vi "Create Queue.vi"(9 "Queue":refnum<class "Queue.lvclass">, 10 "Self Queue Alias":string, 11 "jettl Msg Create Queue in":refnum<class "jettl Msg Create Queue.lvclass">) -> (3 "jettl Msg Create Queue out":refnum<class "jettl Msg Create Queue.lvclass">)   [LabVIEW 2021, in "Create Queue Msg Strategy.lvlib" / "jettl Msg Create Queue.lvclass"]
uses:
  jettl Msg Create Queue.lvclass
  jettl/Queue/Queue.lvclass
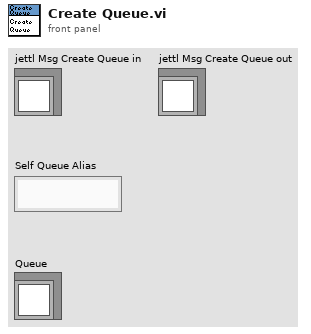
[diagram p1: front panel]
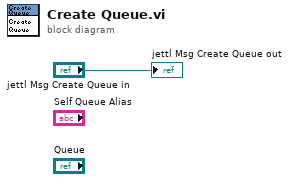
[diagram p0: block diagram]
diagram:
  "jettl Msg Create Queue out" <- "jettl Msg Create Queue in"
